vi "Program_Load_v03.vi"(6 "Time Spin":dbl[unit], 8 "error in (no error)":errorcluster, 9 "Time Start":dbl[unit], 10 "Program Spin Coater":T1(array[cluster]), 11 "SpinCoater in":refnum<class "SpinCoater.lvclass">) -> (0 "error out":errorcluster, 3 "SpinCoater out":refnum<class "SpinCoater.lvclass">)   [LabVIEW 2020, in "SpinCoater.lvclass"]
uses:
  <instrlib>/Classes/SpinCoater/SpinCoater.lvclass
panel:
  out "read buffer":string
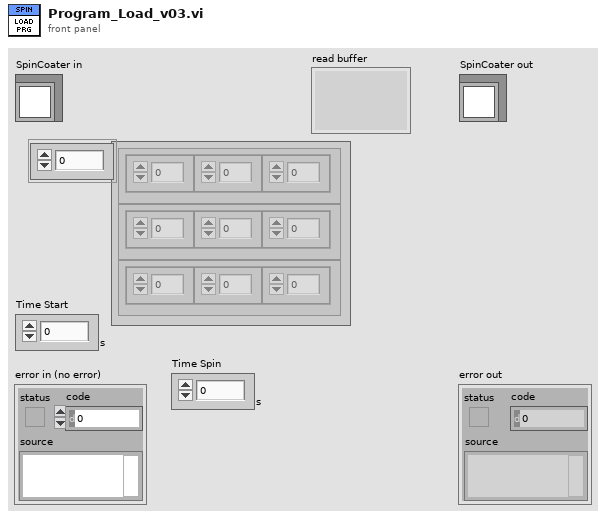
[diagram p1: front panel]
types:
  T1 = cluster{"Speed (rpm)":dbl, "Time (s)":dbl, "Acc (rpm/s)":dbl}[]
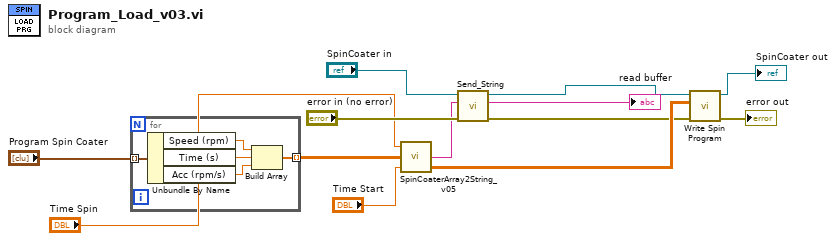
[diagram p0: block diagram]
diagram:
  n1 = for {
    tunnel: "Program Spin Coater" -> [w18] mode=indexing
    tunnel: [w14] -> w5 mode=indexing
    n2 = Unbundle By Name(w18) -> ("Speed (rpm)"=w17:dbl, "Time (s)"=w16:dbl, "Acc (rpm/s)"=w15:dbl)
    n3 = Build Array(w17, w16, w15) -> (w14:dbl[])
  }
  n4 = call <instrlib>:"SpinCoaterArray2String_v05.vi"("Time Start"="Time Start", "Program Spin Coater\nSpeed (rpm)          Time (s)"=w5, "Time Spin"="Time Spin") -> ("Prg Spin Coater small"=w9:dbl[][], "remote control String"=w10:string)  [unwired: 1 in]
  n5 = call-dynamic "Send_String.vi"("error in (no error)"="error in (no error)", "String"=w10, "SpinCoater in"="SpinCoater in") -> ("error out"=w4:errorcluster, "read buffer"=→"read buffer":string, "SpinCoater out"=w2:refnum<class "SpinCoater.lvclass">)  [unwired: 6 in]
  n6 = call-dynamic "Write Spin Program.vi"("error in (no error)"=w4, "Spin Program"=w9, "SpinCoater in"=w2) -> ("error out"=→"error out":errorcluster, "SpinCoater out"=→"SpinCoater out":refnum<class "SpinCoater.lvclass">)  [unwired: 7 in]
